vi "Thorlabs-Stop.vi"(8 "error in (no error)":errorcluster) -> (0 "error out":errorcluster)   [LabVIEW 2020]
uses:
  ECU_SDK/ThorECU.lvlib
  LSM_SDK/ThorConfocal.lvlib
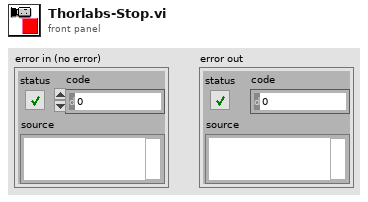
[diagram p1: front panel]
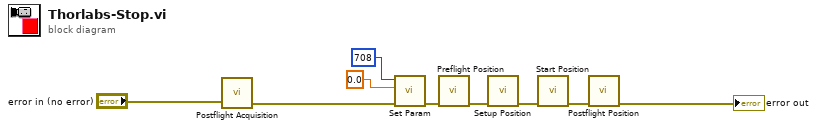
[diagram p0: block diagram]
diagram:
  n1 = call "Postflight Acquisition.vi"("error in (no error)"="error in (no error)") -> ("error out"=w7:errorcluster)  [unwired: 1 in, 2 out]
  n2 = call "Set Param.vi"("error in (no error)"=w7, "param"=0.0, "paramID"=708) -> ("error out"=w3:errorcluster)  [unwired: 7 in, 1 out]
  n3 = call "Preflight Position.vi"("error in (no error)"=w3) -> ("error out"=w4:errorcluster)  [unwired: 9 in, 1 out]
  n4 = call "Setup Position.vi"("error in (no error)"=w4) -> ("error out"=w5:errorcluster)  [unwired: 9 in, 1 out]
  n5 = call "Start Position.vi"("error in (no error)"=w5) -> ("error out"=w6:errorcluster)  [unwired: 9 in, 1 out]
  n6 = call "Postflight Position.vi"("error in (no error)"=w6) -> ("error out"=→"error out":errorcluster)  [unwired: 9 in, 1 out]
